vi "DCS_loc_to_array.vi"(1 "DCS locs in":dbl[](array[numeric])) -> (0 "Array locs out":i32[](array[numeric]))   [LabVIEW 2013]
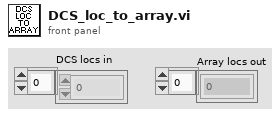
[diagram p1: front panel]
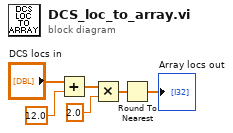
[diagram p0: block diagram]
diagram:
  n1 = Add(x="DCS locs in", y=12.0) -> (x+y=w5:dbl[])
  n2 = Multiply(x=w5, y=2.0) -> (x*y=w3:dbl[])
  n3 = Round To Nearest(number=w3) -> (nearest integer value=→"Array locs out":dbl[])
